vi "uView_fp.insert.vi"(8 "error in (no error)":errorcluster, 10 "subPanel":refnum<vi>, 11 "uView Transport":refnum<class "uTransport_uActor.lvclass">) -> (0 "error out":errorcluster)   [LabVIEW 2023, in "uLib.lvlib" / "uView.lvclass"]
doc: "insert the View into the provided subpanel."
uses:
  uView.lvclass
  uTransport/uTransport_uActor/uTransport_uActor.lvclass
  uData/uData/uData.lvclass
  uData/uData/uData.lvclass/uData.ctl
  uMsg/uMsg/uMsg.lvclass/uMsg.ctl
  uTransport/uTransport_uActor/uTransport_uActor.lvclass/uTransport_uActor.ctl
  uData/uData/Condition Tag Name.vi
  uActor/uActor_SendMsg.vi
  uMsg/uMsg/uMsg Create.vi
  uData/uData/Blank Key Reserved String.vi
  uTransport/uTransport_uActor/uTransport_uActor_SendMsg.vi
  uMsg/uMsg/uMsg Update Timestamp.vi
  uTransport/uTransport/uTransport.lvclass
  uMsg/uMsg/uMsg.lvclass
  uView.lvclass/uView.ctl
  uActor/uActor.lvclass
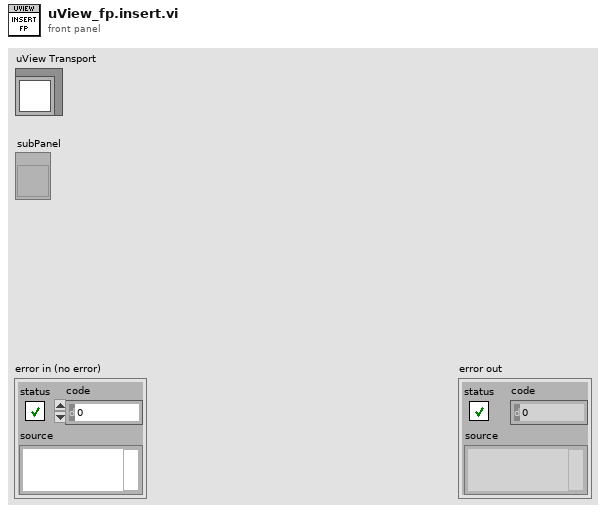
[diagram p1: front panel]
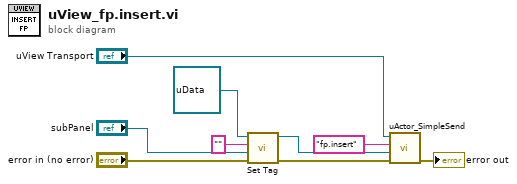
[diagram p0: block diagram]
diagram:
  n1 = call "Set Tag.vi"("error in (no error)"="error in (no error)", "Variant"="subPanel", "tag (case insensitive)"="", "uData in"=refnum<class "uData.lvclass"> refnum) -> ("error out"=w8:errorcluster, "uData out"=w4:refnum<class "uData.lvclass">)  [unwired: 5 in, 1 out]
  n2 = call "uActor_SimpleSend.vi"("error in (no error)"=w8, "Payload"=w4, "Msg"="fp.insert", "uActor Transport"="uView Transport") -> ("error out"=→"error out":errorcluster)  [unwired: 7 in]
